vi "PFI-28000-Card-28144_Get Fault Check Interval.vi"(8 "error in (no error)":errorcluster, 11 "PFI-28000-Card-28144 in":refnum<class "PFI-28000-Card-28144.lvclass">) -> (0 "error out":errorcluster, 2 "Fault Check Interval":i32, 3 "PFI-28000-Card-28144 out":refnum<class "PFI-28000-Card-28144.lvclass">)   [LabVIEW 2017, in "PFI-28000-Card-28144.lvclass"]
uses:
  PFI-28000-Card-28144.lvclass
  C:/wc/07143 Precision Filters 28000 Support/Driver/source/Card/PFI-28000-Card.lvclass
  Channel/PFI-28000-Channel.lvclass
  Utilities/PFI-28000-Utils.lvlib
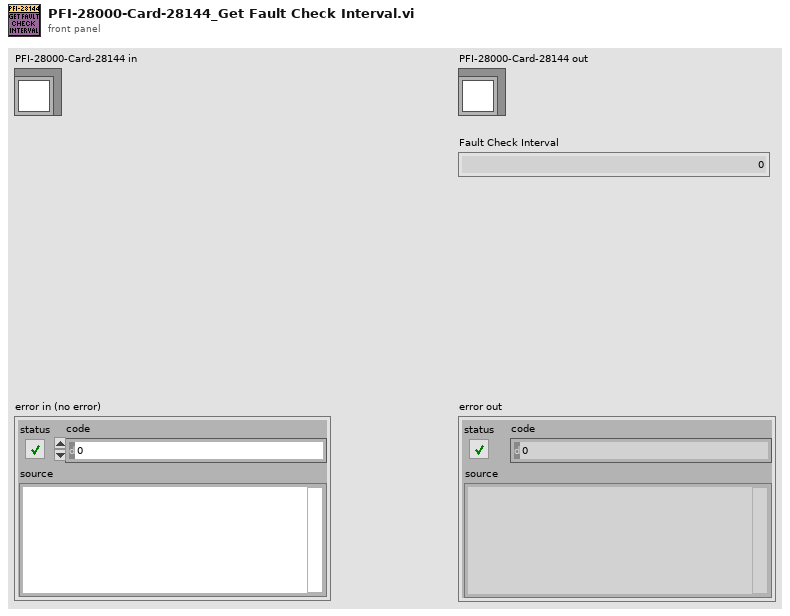
[diagram p1: front panel]
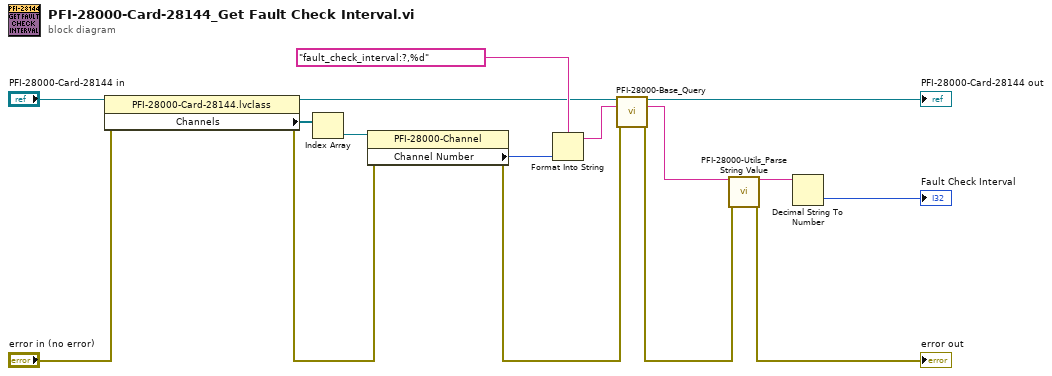
[diagram p0: block diagram]
diagram:
  n1 = property class="PFI-28000-Card-28144.lvclass"(reference="PFI-28000-Card-28144 in", error in="error in (no error)") -> (reference out=w9:refnum<class "PFI-28000-Card-28144.lvclass">, error out=w13:errorcluster, "Channels"=w12:refnum<class "PFI-28000-Channel.lvclass">[])
  n2 = Index Array(array=w12) -> (element=w11:refnum<class "PFI-28000-Channel.lvclass">)  [unwired: 1 in]
  n3 = property class="PFI-28000-Channel"(reference=w11, error in=w13) -> (error out=w7:errorcluster, "Channel Number"=w10:i32)  [unwired: 1 out]
  n4 = Format Into String(format string="fault_check_interval:?,%d" ("empty string"), w10) -> (resulting string=w8:string)  [unwired: 2 in, 1 out]
  n5 = call-dynamic "PFI-28000-Base_Query.vi"("PFI-28000-Base in"=w9, "Command"=w8, "error in (no error)"=w7) -> ("PFI-28000-Base out"=→"PFI-28000-Card-28144 out":refnum<class "PFI-28000-Card-28144.lvclass">, "Response"=w5:string, "error out"=w4:errorcluster)  [unwired: 9 in, 1 out]
  n6 = call "PFI-28000-Utils_Parse String Value.vi"("String"=w5, "error in (no error)"=w4) -> ("String Value"=w2:string, "error out"=→"error out":errorcluster)  [unwired: 11 in, 1 out]
  n7 = Decimal String To Number(string=w2) -> (number=→"Fault Check Interval":i32)  [unwired: 2 in, 1 out]
